vi "AI_StreamingAI_MultipleChannels v5.vi"() -> ()   [LabVIEW 2013]
uses:
  <userlib>/DAQNavi Polymorphic VI/create/DAQNavi Create Channel(AI-Voltage).vi
  <userlib>/DAQNavi Polymorphic VI/configure/timing/DAQNavi Timing(Convert Clock).vi
  <userlib>/DAQNavi Polymorphic VI/configure/DAQNavi Get Property/AI/DAQNaviGet_AI_ConvertClock_Rate.vi
  <userlib>/DAQNavi Polymorphic VI/read/DAQNavi Read (Analog 1D Wfm NChan NSamp).vi
panel:
  out "error out":errorcluster
  out "Waveform Graph":waveform(dbl)[](graph)
  out "value range":string="+/- 5 V" caption="property value"
  out "physical channels":string="DemoDevice,BID#0/ai0:1" caption="property value"
  in  "number of samples per channel to read":u32=1000
  in  "samples per channel":i32=1024
  out "actual convert rate":dbl
  in  "convert clock rate":dbl=1000.0
  out "overrun count":i32
  in  "stop":bool
  # "Please modify physical channels and value range in Channel Parameters\nthrough DAQNavi Property Assistant VI  in block diagram."
  # "Channel Parameters"
  # "Timing Parameters"
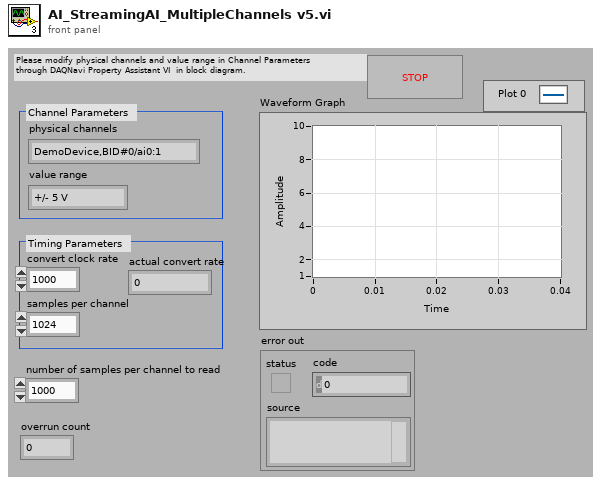
[diagram p1: front panel]
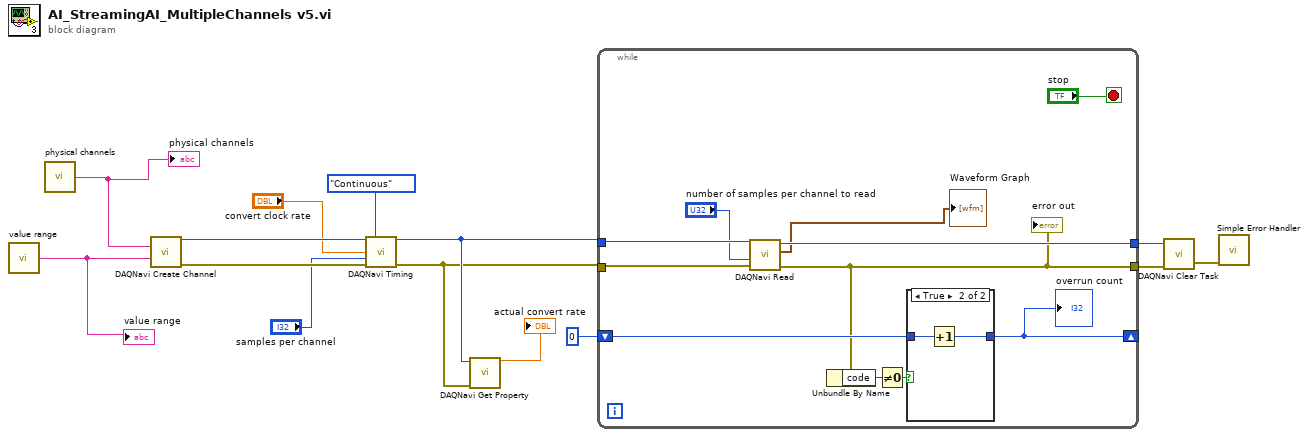
[diagram p0: block diagram]
diagram:
  n1 = call "value range"() -> ("property value"=w3:string)  [unwired: 1 out]
  "value range" <- w3
  n2 = call "physical channels"() -> ("property value"=w4:string)  [unwired: 1 out]
  "physical channels" <- w4
  n3 = call-poly <userlib>:"DAQNavi Create Channel.vi"("physical channels"=w4, "value range"=w3) -> ("task out"=w13:i32, "error out"=w12:errorcluster)  [unwired: 3 in, 9 out]
  n4 = call-poly <userlib>:"DAQNavi Timing.vi"("task in"=w13, "sample mode"=enum16{"Finite", "Continuous"}."Continuous", "rate"="convert clock rate", "samples per channel"="samples per channel", "error in (no error)"=w12) -> ("task out"=w8:i32, "error out"=w7:errorcluster)  [unwired: 1 in, 8 out]
  n5 = call-poly <userlib>:"DAQNavi Get Property.vi"("error in (no error)"=w7, "task in"=w8) -> ("rate"=→"actual convert rate":dbl)  [unwired: 9 out]
  n6 = while {
    tunnel: w8 -> [w24]
    tunnel: w7 -> [w25]
    shift-right: [w20] -> _
    shift-left: 0 -> [w21]
    tunnel: [w18] -> w2
    tunnel: [w17] -> w1
    stop <- "stop" stop-if-true
    n7 = call-poly <userlib>:"DAQNavi Read.vi"("error in (no error)"=w25, "number of samples per channel to read"="number of samples per channel to read", "task in"=w24) -> ("error out"=w17:errorcluster, "data"=→"Waveform Graph":waveform(dbl)[], "task out"=w18:i32)  [unwired: 1 in, 5 out]
    "error out" <- w17
    n8 = Unbundle By Name(w17) -> ("code"=w23:i32)
    n9 = Not Equal To 0?(x=w23) -> (x != 0?=w22:bool)
    n10 = case shown="True" w22 {
      tunnel: w21 -> [w26 w28]
      tunnel: [w26 w27] -> w20
      frame False {
      }
      frame True {
        n11 = Increment(x=w28) -> (x+1=w27:i32)
      }
    }
    "overrun count" <- w20
  }
  n12 = call <userlib>:"DAQNavi Clear Task.vi"("error in (no error)"=w1, "task in"=w2) -> ("error out"=w14:errorcluster)  [unwired: 1 out]
  n13 = call <vilib>:"Simple Error Handler.vi"("error in (no error)"=w14) -> ()  [unwired: 2 in, 7 out]
